vi "Write String.vi"(8 "error in (no error)":errorcluster, 10 "String":string, 11 "Clock Time in":refnum<class "Clock Time.lvclass">) -> (0 "error out":errorcluster, 3 "Clock Time out":refnum<class "Clock Time.lvclass">)   [LabVIEW 2024, in "Clock Time.lvclass"]
doc: "Clock TIme.lvclass:Read Config.vi\n\nThis VI does not do anything, but is only for compatibility with the Bus class. The \"Clock Time\" class does not support writing anything.\n\nInstrument Communication Module Version 1.0\nAugust, 2017 Original Code Consulting David Thomson\n www.originalcode.com"
uses:
  Clock Time.lvclass
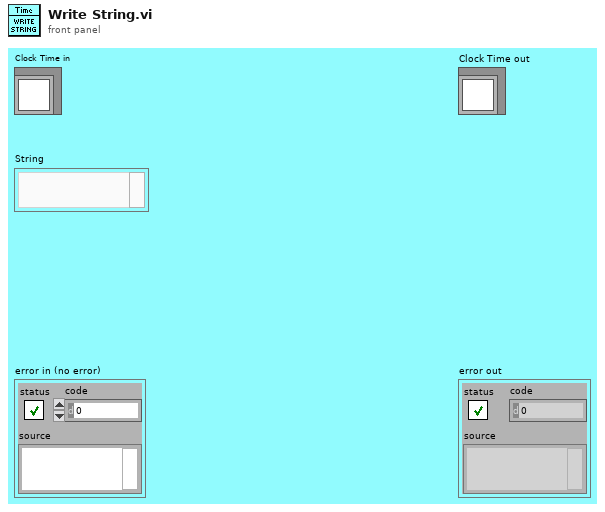
[diagram p1: front panel]
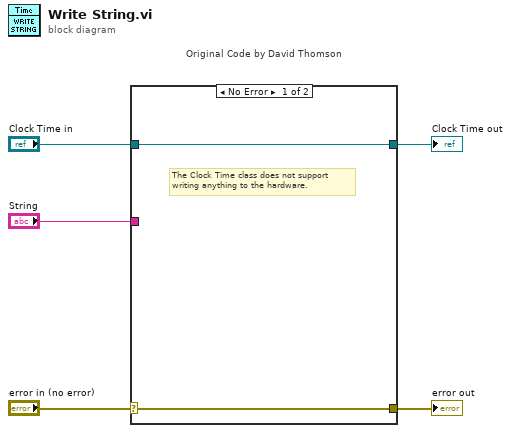
[diagram p0: block diagram]
diagram:
  n1 = case "Original Code by David Thomson" shown="No Error" "error in (no error)" {
    selector: "error in (no error)" -> [w6 w9]
    tunnel: [w6 w9] -> w4
    tunnel: [w7 w8] -> w2
    tunnel: "Clock Time in" -> [w7 w8]
    tunnel: "String" -> [_ _]
    frame No Error {
      # "The Clock Time class does not support\nwriting anything to the hardware."
    }
    frame Error {
    }
  }
  "error out" <- w4
  "Clock Time out" <- w2
